vi "UpdateConsole.vi"(7 "JPG":refnum<vi>, 8 "from last time raw":string, 9 "New Text":string, 11 "Console":string) -> (0 "Left over raw":string, 1 "left over fixed":string, 2 "LastFullLine":string, 3 "Console Out":string, 4 "cursor out":i32, 5 "lines":string[](array[string]))   [LabVIEW 2022 SP3]
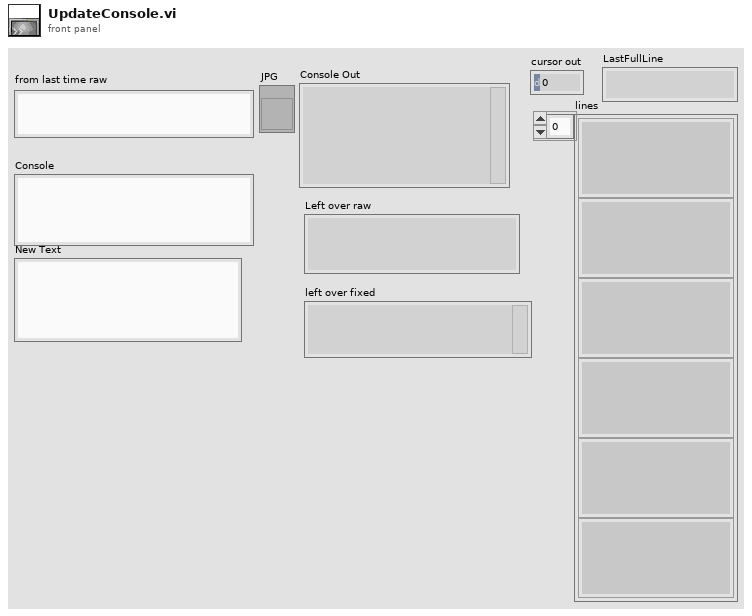
[diagram p1: front panel]
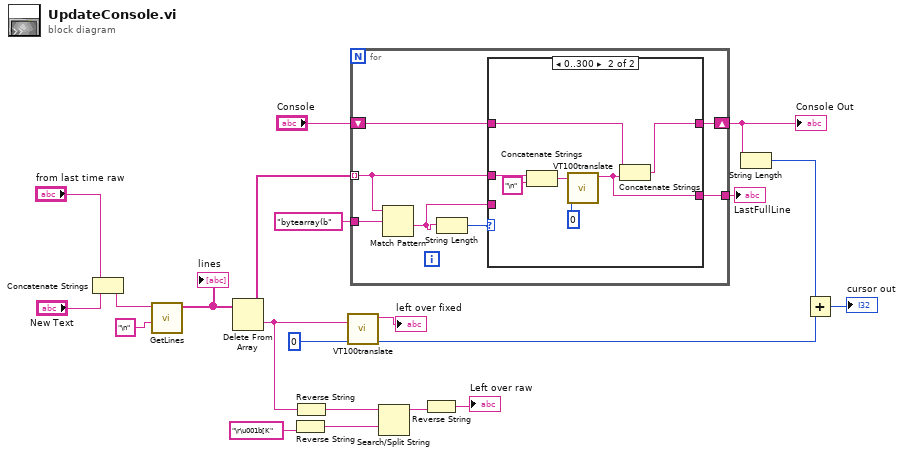
[diagram p0: block diagram]
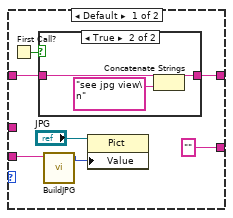
[diagram p2: hidden frame]
diagram:
  n1 = Concatenate Strings("from last time raw", "New Text") -> (w11:string)
  n2 = call "GetLines.vi"("delimiter"="\n", "String"=w11) -> ("Array"=w10:string[])  [unwired: 9 in]
  "lines" <- w10
  n3 = Delete From Array(array=w10) -> (deleted portion=w9:string, array with subset deleted=w17:string[])  [unwired: 2 in]
  n4 = Reverse String(1:"\r\u001b[K" ("New Text")) -> (0:w5:string)
  n5 = Reverse String(1:w9) -> (0:w6:string)
  n6 = call "VT100translate.vi"("cursor in"=0, "Text"=w9) -> ("cursor out"=w14:i32, "Console fixed"=→"left over fixed":string)  [unwired: 8 in]
  n7 = for {
    shift-right: [w28] -> w16
    shift-left: "Console" -> [w27]
    tunnel: w17 -> [w25] mode=indexing
    tunnel: [w26] -> w2
    tunnel: "bytearray(b" ("regular expression") -> [w22]
    n8 = Match Pattern(string=w25, regular expression=w22) -> (after substring=w23:string)  [unwired: 1 in, 3 out]
    n9 = String Length(string=w23) -> (length=w24:i32)
    n10 = case shown="0..300" w24 {
      tunnel: [w31 w46] -> w28
      tunnel: w27 -> [w30 w45]
      tunnel: ["" ("Console fixed") w41] -> w26
      tunnel: w25 -> [_ w40]
      tunnel: w23 -> [w34 _]
      frame Default {
        n11 = First Call?() -> (First Call?: T/F=w29:bool)
        n12 = case shown="True" w29 {
          tunnel: [w36 w39] -> w31
          tunnel: w30 -> [w36 w38]
          frame False {
          }
          frame True {
            n13 = Concatenate Strings(w38, "see jpg view\n" ("Console fixed")) -> (w39:string)
          }
        }
        n14 = call "BuildJPG.vi"("image"=w34) -> ("new picture"=w32:picture)  [unwired: 10 in]
        n15 = property class="Pict"(reference="JPG", "Value"=w32) -> ()  [unwired: 1 in, 2 out]
      }
      frame 0..300 {
        n16 = Concatenate Strings(w40, "\n" ("regular expression")) -> (w43:string)
        n17 = call "VT100translate.vi"("cursor in"=0, "Text"=w43) -> ("Console fixed"=w41:string)  [unwired: 8 in, 1 out]
        n18 = Concatenate Strings(w45, w41) -> (w46:string)
      }
    }
  }
  "Console Out" <- w16
  "LastFullLine" <- w2
  n19 = Search/Split String(string=w6, search string/char (-)=w5) -> (substring before match=w8:string)  [unwired: 1 in, 2 out]
  n20 = Reverse String(1:w8) -> (0:→"Left over raw":string)
  n21 = String Length(string=w16) -> (length=w15:i32)
  n22 = Add(x=w15, y=w14) -> (x+y=→"cursor out":i32)
